vi "0002-03.vi"(9 "Pas":dbl, 10 "x_deb":dbl, 11 "Nb":u32) -> (3 "sér. (s)":T1)   [LabVIEW 2010, in "lv_01.lvlib"]
doc: "La série est générée à partie des 3 grandeurs scalaires x_deb, Nb et Pas."
uses:
  lv_01.lvlib
  do_serie-c.ctl
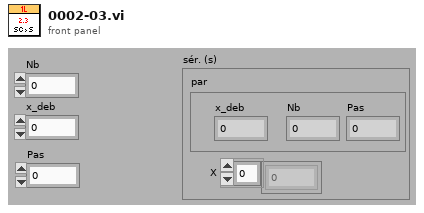
[diagram p1: front panel]
types:
  T1 = typedef "lv_01.lvlib/do_serie-c.ctl" = cluster{"X":dbl[], "par":cluster{"x_deb":dbl, "Pas":dbl, "Nb":dbl}}
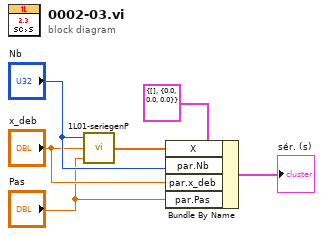
[diagram p0: block diagram]
diagram:
  n1 = call "1L01-seriegenP.vi"("Pas"="Pas", "x_deb"="x_deb", "Nb"="Nb") -> ("X"=w5:dbl[])
  n2 = Bundle By Name(cluster=T1 {"X"=[], "par"={"x_deb"=0.0, "Pas"=0.0, "Nb"=0.0}} ("sér. (s) 2"), "X"=w5, "par.Nb"="Nb", "par.x_deb"="x_deb", "par.Pas"="Pas") -> (→"sér. (s)":T1)
